vi "readBaseFASettings.vi"(8 "error in (no error)":errorcluster, 11 "Boot in":refnum<class "Boot.lvclass">) -> (0 "error out":errorcluster, 2 "BaseForceActuatorSettings":T1, 3 "Boot out":refnum<class "Boot.lvclass">)   [LabVIEW 2016, in "Boot.lvclass"]
uses:
  Boot.lvclass
  DataTypes/Settings/Base/BaseFASettings.ctl
  Common_RT_FAILC/DataTypes/FATimings.ctl
  Boot.lvclass/Boot.ctl
  Settings/Settings/Setting.lvclass
  Common_RT_FAILC/RTFAILC.lvlib
  DataTypes/Settings/M1M3SupportSettings.lvlib
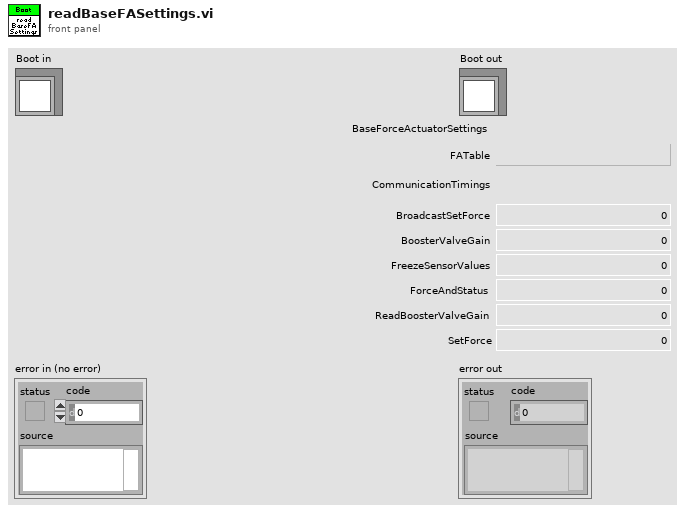
[diagram p1: front panel]
types:
  T1 = typedef "M1M3SupportSettings.lvlib/BaseFASettings.ctl" = cluster{"CommunicationTimings":T2, "FATable":path}
  T2 = typedef "RTFAILC.lvlib/FATimings.ctl" = cluster{"BroadcastSetForce":u32, "BoosterValveGain":u32, "FreezeSensorValues":u32, "ForceAndStatus":u32, "ReadBoosterValveGain":u32, "SetForce":u32}
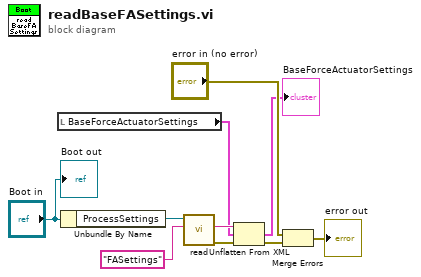
[diagram p0: block diagram]
diagram:
  n1 = local read "BaseForceActuatorSettings"() -> (w7:T1)
  n2 = Unbundle By Name("Boot in") -> ("ProcessSettings"=w10:refnum<class "Setting.lvclass">)
  n3 = call-dynamic "read.vi"("Name"="FASettings", "BaseSetting in"=w10) -> ("error out"=w5:errorcluster, "XML"=w8:string)  [unwired: 6 in, 2 out]
  n4 = Unflatten From XML(xml string=w8, type=w7, error in (no error)=w5) -> (value=→"BaseForceActuatorSettings":T1, error out=w2:errorcluster)
  n5 = Merge Errors("error in (no error)", w2) -> (→"error out":errorcluster)
  "Boot out" <- "Boot in"
